vi "nanomsg_close.vi"(3 "error in":errorcluster, 5 "socket":refnum<class "nanomsg_socket.lvclass">) -> (0 "error out":errorcluster)   [LabVIEW 2014, in "nanomsg.lvlib" / "nanomsg_socket.lvclass"]
doc: "Signal that the socket is no longer required and to free it once pending operations are finished.\n\nNote that this is a <b>non-blocking</b> function and the socket is not necessarily closed when it returns. Any operations pending will be completed before the socket is closed and port freed. To interrupt blocking calls use ctx_destroy.\n\nDetailed API documentation: http://nanomsg.org/documentation.html"
uses:
  nanomsg_socket.lvclass
  nanomsg_socket.lvclass/nanomsg_socket.ctl
  <vilib>/Utility/error.llb/Error Cluster From Error Code.vi
  nanomsg.lvlib
panel:
  # "NN"
  # "labview"
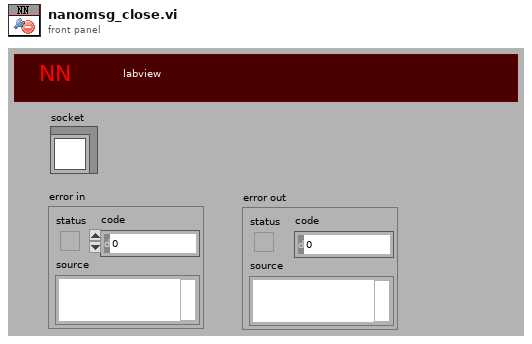
[diagram p1: front panel]
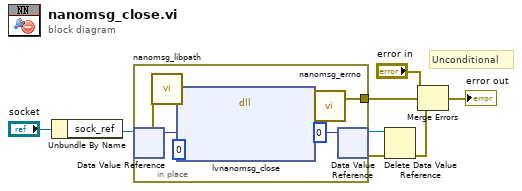
[diagram p0: block diagram]
diagram:
  # "Unconditional"
  n1 = Unbundle By Name("socket") -> ("sock_ref"=w7:refnum<data-value>)
  n2 = in-place {
    in-place-border: [w14] -> w3
    n3 = in-place-dvr #1(w7) -> (w12:u64, w9:errorcluster)
    n4 = call "nanomsg_libpath.vi"() -> ("path"=w10:path)
    n5 = dll-call lib="?" fn="lvnanomsg_close" ("libzmq.dll:zmq_close")(path in=w10, error in=w9, "sock_obj"=w12, "flags"=0 ("kill")) -> (error out=w15:errorcluster, "return"=w16:i32)  [unwired: 3 in, 1 out]
    n6 = call "nanomsg_errno.vi"("retval"=w16, "error in"=w15) -> ("error out"=w14:errorcluster)  [unwired: 1 out]
    n7 = in-place-dvr #1(u64 0 ("data value")) -> (w5:refnum<data-value>, w6:errorcluster)
  }
  n8 = Delete Data Value Reference(data value reference=w5, error in=w6) -> (error out=w1:errorcluster)  [unwired: 1 out]
  n9 = Merge Errors("error in", w3, w1) -> (→"error out":errorcluster)
